vi "保存数据.vi"() -> ()   [LabVIEW 2018]
uses:
  <vilib>/Utility/file.llb/Write Delimited Spreadsheet (DBL).vi
panel:
  in  "X":i32
  in  "Y":i32
  in  "缓冲区长度":u32=60000
  in  "采集点数":i32
  in  "VISA资源":refnum<visa-resource-name>
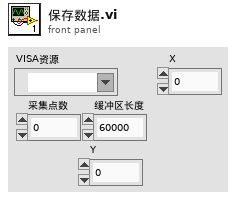
[diagram p1: front panel]
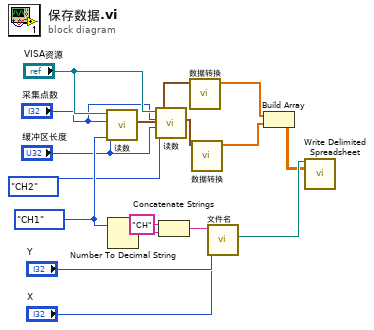
[diagram p0: block diagram]
diagram:
  w16 = enum16{"CH1", "CH2"}."CH1" ("通道选择")
  n1 = call "读数.vi"("error in"=w16, 9:"缓冲区长度", 10:"采集点数", "设置"="VISA资源") -> ("触发信号"=w12:waveform(dbl))  [unwired: 5 in, 2 out]
  n2 = Number To Decimal String(number=w16) -> (decimal integer string=w15:string)  [unwired: 1 in]
  n3 = call "读数.vi"("error in"=enum16{"CH1", "CH2"}."CH2" ("通道选择"), 9:"缓冲区长度", 10:"采集点数", "设置"="VISA资源") -> ("触发信号"=w4:waveform(dbl))  [unwired: 5 in, 2 out]
  n4 = Concatenate Strings("CH" ("字符串"), w15) -> (w13:string)
  n5 = call "数据转换.vi"("数据输入"=w12) -> ("波形数组"=w3:dbl[])  [unwired: 10 in]
  n6 = call "数据转换.vi"("数据输入"=w4) -> ("波形数组"=w2:dbl[])  [unwired: 10 in]
  n7 = call "文件名.vi"("第n个文件"="X", "文件类型"="Y", 11:w13) -> ("添加的路径"=w9:path)  [unwired: 8 in]
  n8 = Build Array(w3, w2) -> (w1:dbl[][])
  n9 = call-poly <vilib>:"Write Delimited Spreadsheet.vi"("file path (dialog if empty)"=w9, "2D data"=w1) -> ()  [unwired: 12 in, 2 out]
